vi "read.vi"(8 "error in (no error)":errorcluster, 11 "CNT90 in":refnum<class "CNT90.lvclass">) -> (0 "error out":errorcluster, 2 "medicion":dbl, 3 "CNT90 out":refnum<class "CNT90.lvclass">)   [LabVIEW 2019, in "CNT90.lvclass"]
uses:
  CNT90.lvclass
  CNT90.lvclass/CNT90.ctl
  <instrlib>/Pendulum CNT90/Public/Data/Read Measurement (Single).vi
  <instrlib>/Pendulum CNT90/Pendulum CNT90.lvlib
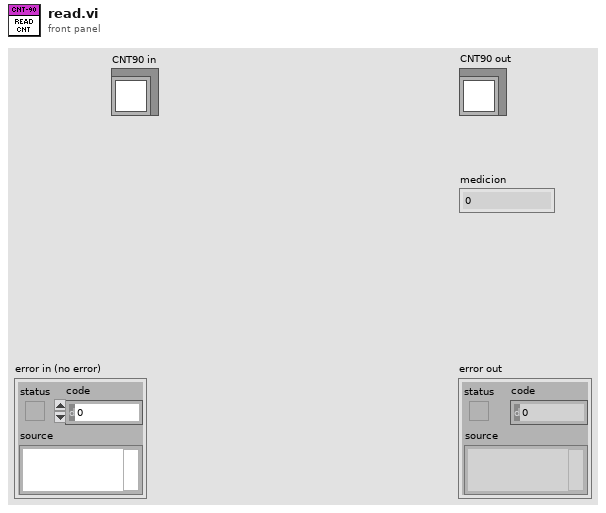
[diagram p1: front panel]
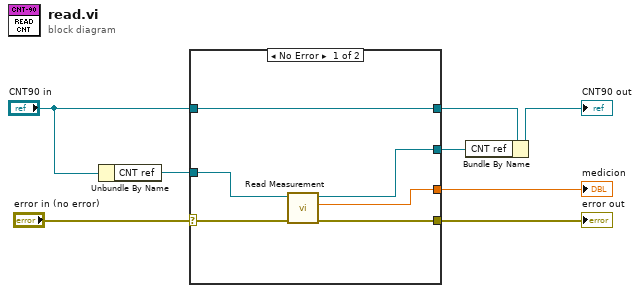
[diagram p0: block diagram]
diagram:
  n1 = Unbundle By Name("CNT90 in") -> ("CNT ref"=w3:refnum<visa-resource-name>)
  n2 = case shown="No Error" "error in (no error)" {
    selector: "error in (no error)" -> [w12 w17]
    tunnel: [w11 w17] -> w7
    tunnel: [w14 w16] -> w6
    tunnel: "CNT90 in" -> [w14 w16]
    tunnel: w3 -> [w13 w15]
    tunnel: [w10 _] -> w5
    tunnel: [w9 w15] -> w1
    frame No Error {
      n3 = call-poly <instrlib>:"Read Measurement.vi"("error in (no error)"=w12, "VISA resource name"=w13) -> ("error out"=w11:errorcluster, "Measurement"=w10:dbl, "VISA resource name out"=w9:refnum<visa-resource-name>)  [unwired: 7 in]
    }
    frame Error {
    }
  }
  "error out" <- w7
  "medicion" <- w5
  n4 = Bundle By Name(cluster=w6, "CNT ref"=w1) -> (→"CNT90 out":refnum<class "CNT90.lvclass">)
